vi "BartelsMPXMessageLoop.vi"(8 "Error In":errorcluster, 11 "CommunicationRefs":T1) -> (0 "Error Out":errorcluster)   [LabVIEW 2015]
uses:
  TypeDefs/CommunicationRefs.ctl
  TypeDefs/MessageCluster.ctl
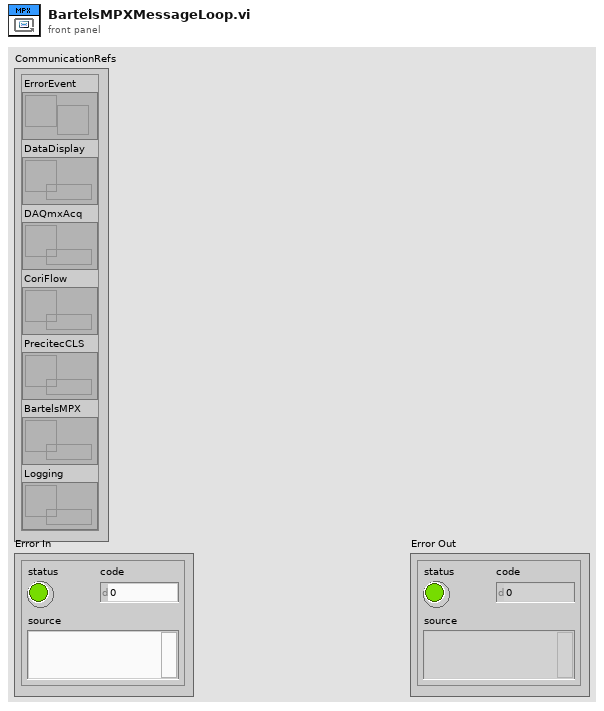
[diagram p1: front panel]
types:
  T1 = typedef "CommunicationRefs.ctl" = cluster{"ErrorEvent":refnum<user-event>, "DataDisplay":refnum<queue>, "DAQmxAcq":refnum<queue>, "CoriFlow":refnum<queue>, "PrecitecCLS":refnum<queue>, "BartelsMPX":refnum<queue>, "Logging":refnum<queue>}
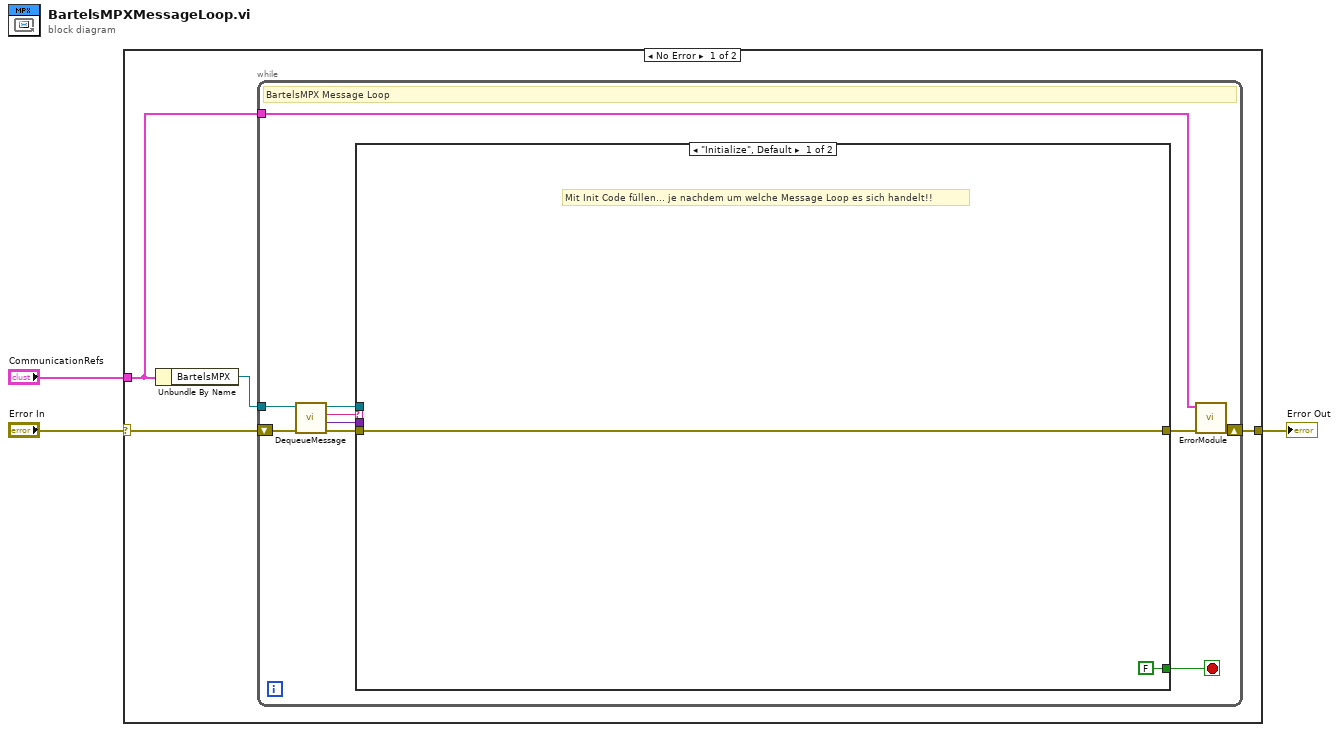
[diagram p0: block diagram]
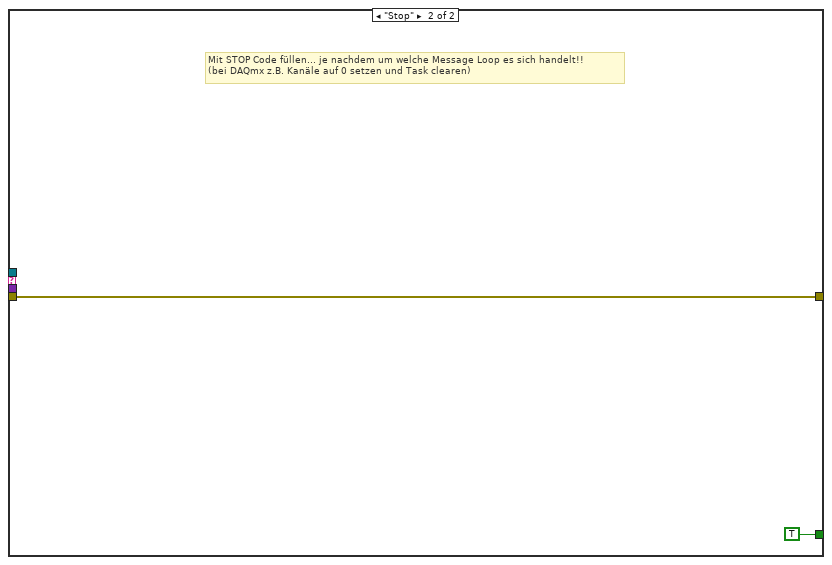
[diagram p2: hidden frame]
diagram:
  n1 = case shown="No Error" "Error In" {
    selector: "Error In" -> [w6 w22]
    tunnel: [w5 w22] -> w2
    tunnel: "CommunicationRefs" -> [w4 _]
    frame No Error {
      n2 = Unbundle By Name(w4) -> ("BartelsMPX"=w7:refnum<queue>)
      n3 = while {
        tunnel: w7 -> [w17]
        tunnel: w4 -> [w9]
        shift-right: [w11] -> w5
        shift-left: w6 -> [w16]
        stop <- w8 stop-if-true
        # "BartelsMPX Message Loop"
        n4 = call "DequeueMessage.vi"("error in (no error)"=w16, "MessageQueue"=w17) -> ("error out"=w12:errorcluster, "MessageData"=w13:variant, "Message"=w14:string, "dupMessageQueue"=w15:refnum<queue>)  [unwired: 6 in]
        n5 = case shown="\"Initialize\", Default" w14 {
          tunnel: w15 -> [_ _]
          tunnel: w13 -> [_ _]
          tunnel: w12 -> [w19 w21]
          tunnel: [w19 w21] -> w10
          tunnel: [FALSE TRUE] -> w8
          frame "Initialize", Default {
            # "Mit Init Code füllen... je nachdem um welche Message Loop es sich handelt!!"
          }
          frame "Stop" {
            # "Mit STOP Code füllen... je nachdem um welche Message Loop es sich handelt!!\n(bei DAQmx z.B. Kanäle auf 0 setzen und Task clearen)"
          }
        }
        n6 = call "ErrorModule.vi"("Error In"=w10, "CommunicationRefs"=w9) -> ("Error Out"=w11:errorcluster)  [unwired: 9 in]
      }
    }
    frame Error {
    }
  }
  "Error Out" <- w2
